vi "CreateDependencyItemRuleObject.vi"(8 "error in (no error)":errorcluster, 9 "Parent Layer":string, 11 "delimited name":string) -> (0 "error out":errorcluster, 3 "IDependencyItemRule":refnum<class "IDependencyItemRule.lvclass">)   [LabVIEW 2020, in "LabVIEWObjectFactory.lvlib"]
uses:
  LabVIEWObjectFactory.lvlib
  LabVIEWObjectInterfaces/IDependencyItemRule/IDependencyItemRule.lvclass
  LabVIEWContainers/CDependencyItemRule/CDependencyItemRule.lvclass
  E:/Repos/LVDependencyInspector/src/LabVIEWObjectInterfaces/IDependencyItemRule/IDependencyItemRule.lvclass
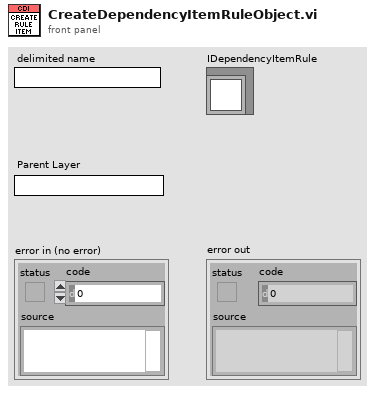
[diagram p1: front panel]
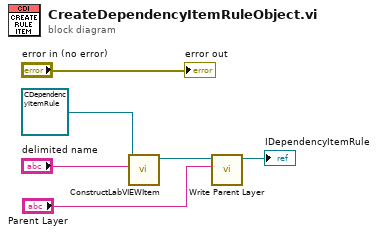
[diagram p0: block diagram]
diagram:
  n1 = call-dynamic "ConstructLabVIEWItem.vi"("Qualified name"="delimited name", "CLabVIEWItem in"=refnum<class "CDependencyItemRule.lvclass"> refnum ("DGML_Generator_Helper.lvlib:CDependencyItemRule.lvclass")) -> ("CLabVIEWItem out"=w3:refnum<class "CDependencyItemRule.lvclass">)  [unwired: 8 in, 1 out]
  n2 = call-dynamic "Write Parent Layer.vi"("Parent Layer"="Parent Layer", "CDependencyItemRule in"=w3) -> ("CDependencyItemRule out"=→"IDependencyItemRule":refnum<class "CDependencyItemRule.lvclass">)  [unwired: 9 in]
  "error out" <- "error in (no error)"
